vi "Project.vi"() -> ()   [LabVIEW 2023]
uses:
  System.Windows.Forms
  <vilib>/Utility/file.llb/Read Delimited Spreadsheet (string).vi
  <instrlib>/Agilent N934X Series/Public/Configure/Measurement/Configure Measurement (Reflection Measurement).vi
  <instrlib>/Agilent N934X Series/Public/Configure/Measurement/Configure Measurement (Reflection Measurement - DTF).vi
  <instrlib>/Agilent N934X Series/Public/Configure/Configure Frequency (Reflection Measurement - Start Stop).vi
  <vilib>/Utility/file.llb/Write Delimited Spreadsheet (string).vi
  <instrlib>/Agilent N934X Series/Agilent N934X Series.lvlib
panel:
  in  "VISA resource name":refnum<visa-resource-name>
  out "loop#":i32
  in  "jkjk":bool
  out "jkjk":string
  out "jkjk":string
  out "jkjk":string
  in  "jkjk":bool
  in  "Tab Control":T1(tab)
  in  "?":bool
  out "?":string
  out "Step:":i32
  in  "Length of Cable (ft)":dbl=5.0
  in  "?":refnum<k24>(container)
  out "Section:":string
  # "VSWR and Distance to Fault Test"
  # "For a single carrier"
  # "(LBand TX)  +  LBand RX = 2475 MHz"
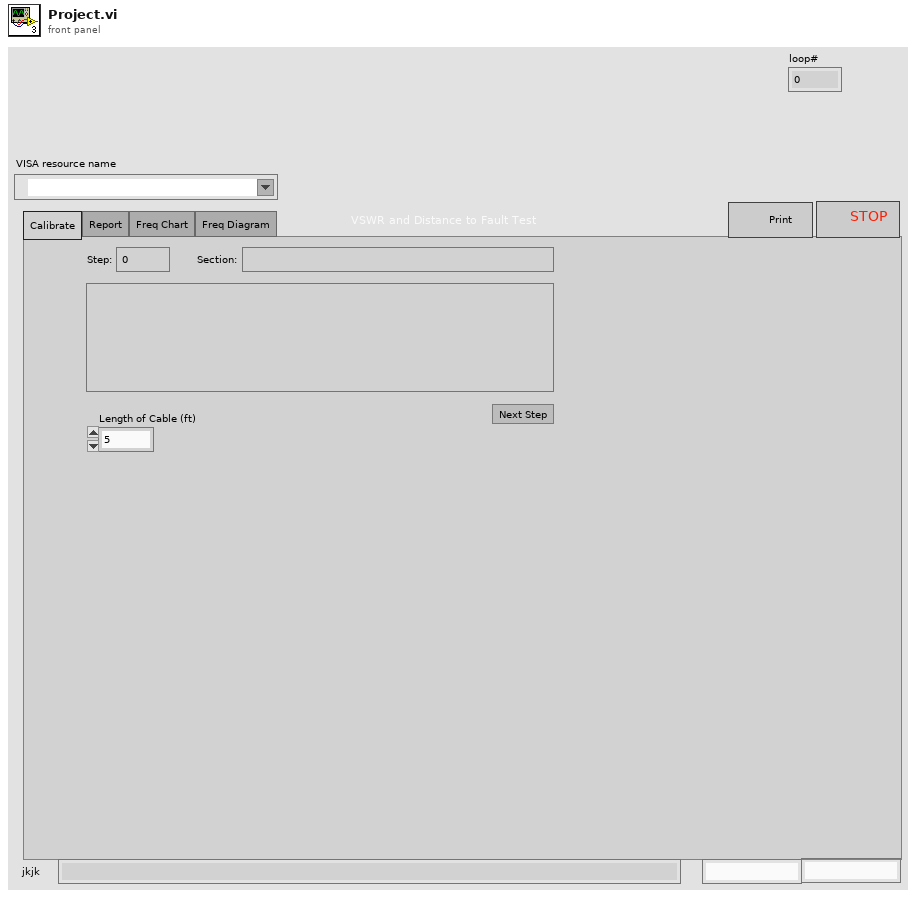
[diagram p1: front panel]
types:
  T1 = enum32{"Calibrate", "Report", "Freq Chart", "Freq Diagram"}
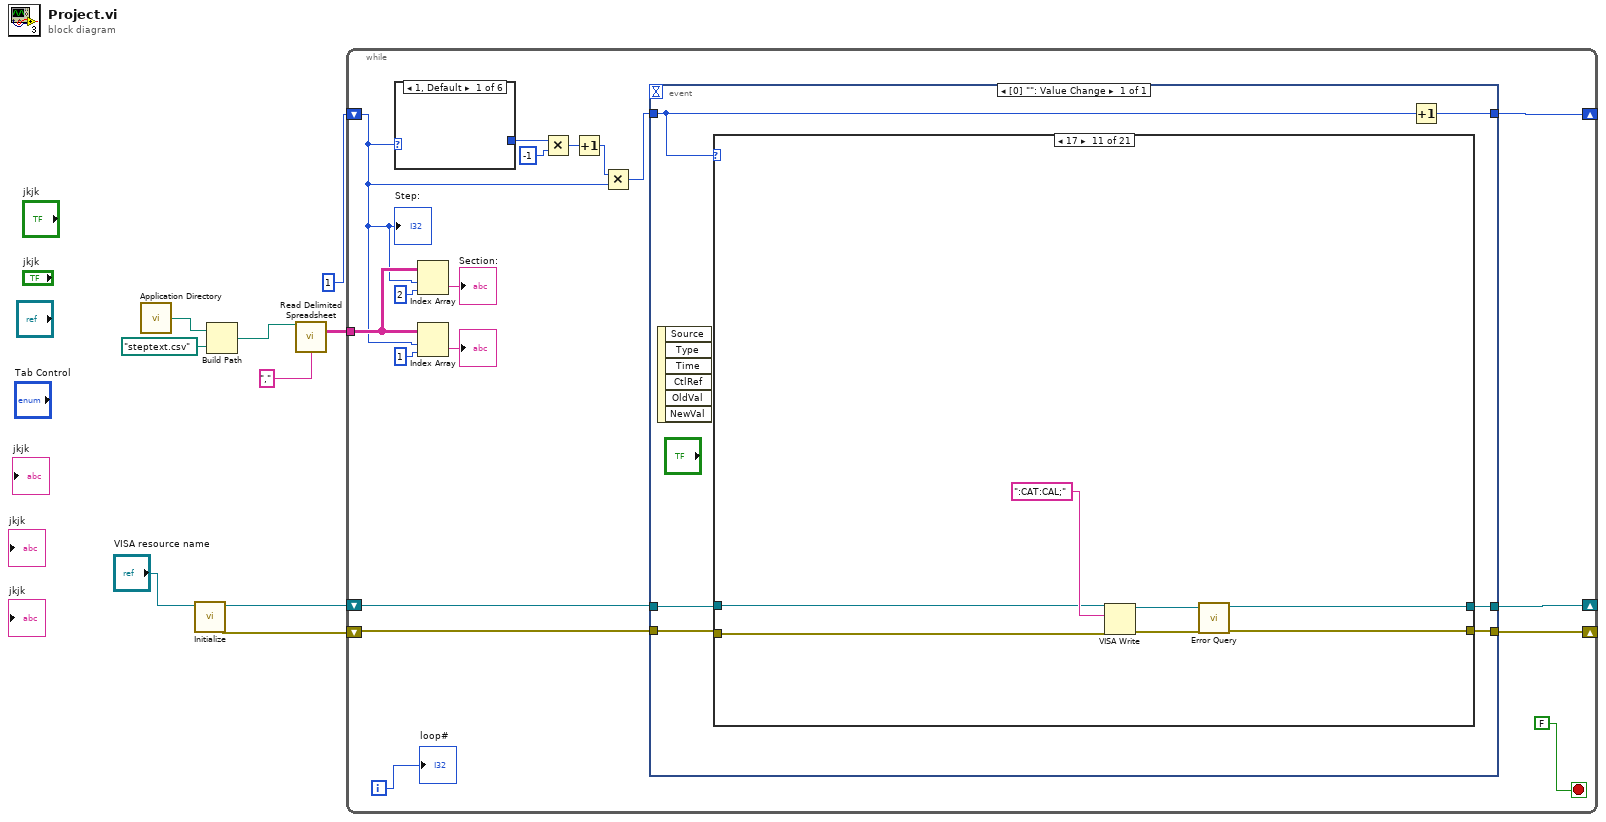
[diagram p0: block diagram]
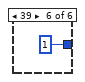
[diagram p6: hidden frame]
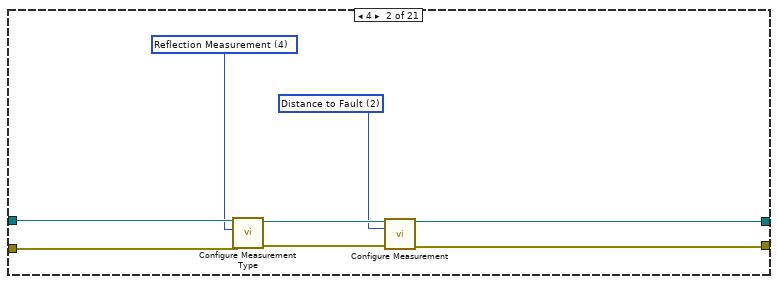
[diagram p8: hidden frame]
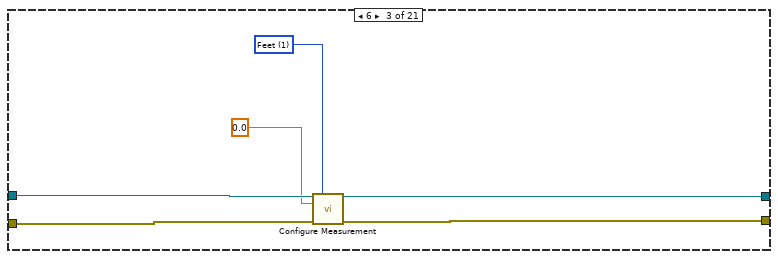
[diagram p9: hidden frame]
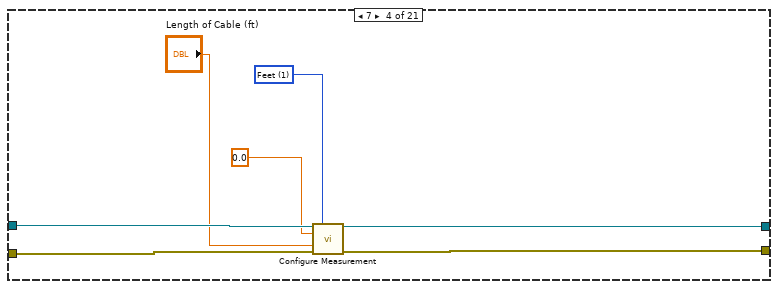
[diagram p10: hidden frame]
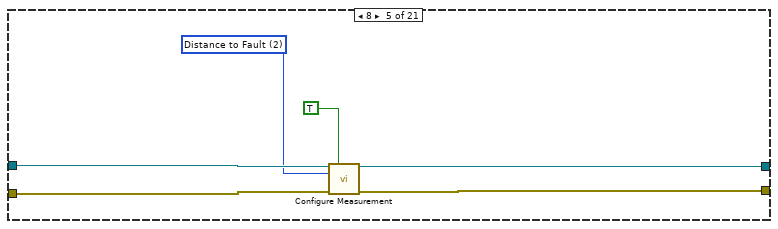
[diagram p11: hidden frame]
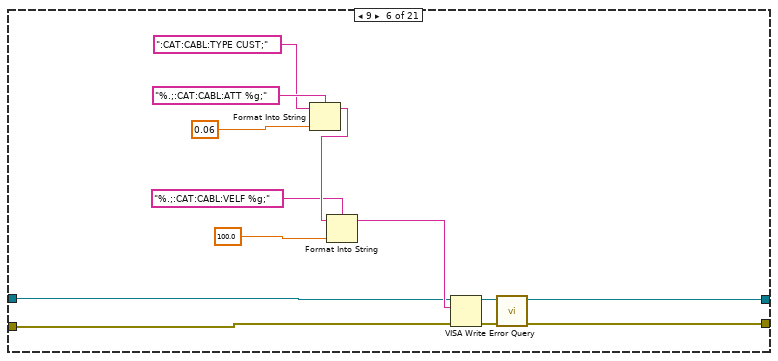
[diagram p12: hidden frame]
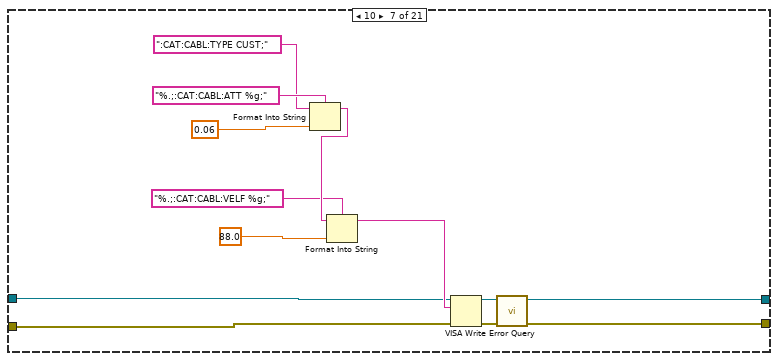
[diagram p13: hidden frame]
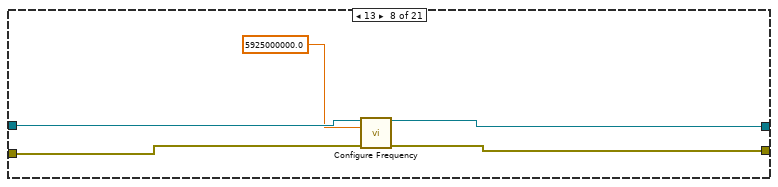
[diagram p14: hidden frame]
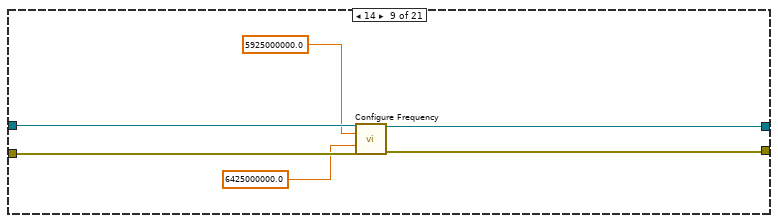
[diagram p15: hidden frame]
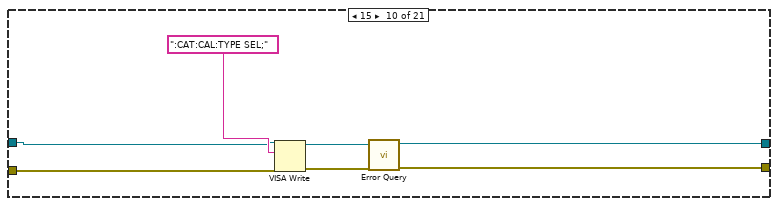
[diagram p16: hidden frame]
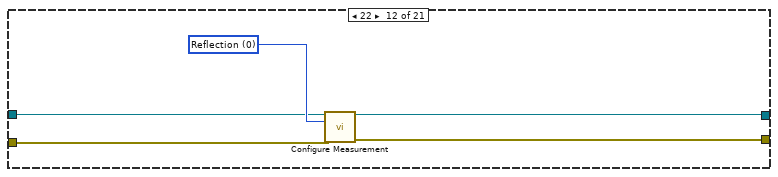
[diagram p17: hidden frame]
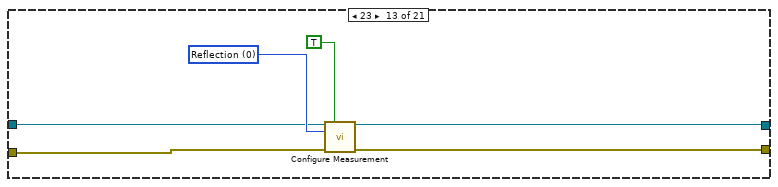
[diagram p18: hidden frame]
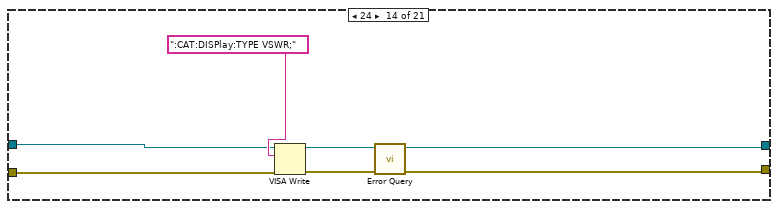
[diagram p19: hidden frame]
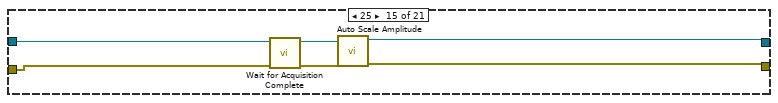
[diagram p20: hidden frame]
diagram:
  n1 = call <vilib>:"Application Directory.vi"() -> ("Application Directory"=w6:path)
  n2 = call <instrlib>:"Initialize.vi"("VISA resource name"="VISA resource name") -> ("error out"=w1:errorcluster, "VISA resource name out"=w2:refnum<visa-resource-name>)  [unwired: 9 in]
  n3 = Build Path(base path=w6, name or relative path=path "steptext.csv") -> (appended path=w4:path)
  n4 = call-poly <vilib>:"Read Delimited Spreadsheet.vi"("file path (dialog if empty)"=w4, "delimiter (\\t)"="," ("delimiter (\\t)")) -> ("all rows"=w7:string[][])  [unwired: 8 in, 5 out]
  n5 = while {
    shift-right: [w25] -> _
    shift-left: 1 -> [w15]
    tunnel: w7 -> [w17]
    shift-right: [w13] -> _
    shift-left: w2 -> [w11]
    shift-right: [w12] -> _
    shift-left: w1 -> [w10]
    i -> [w14]
    stop <- FALSE stop-if-true
    n6 = case shown="1, Default" w15 {
      tunnel: [_ _ _ _ _ 1] -> w24
      frame 1, Default {
      }
      frame 2 {
      }
      frame 3 {
      }
      frame 4 {
      }
      frame 5 {
      }
      frame 39 {
      }
    }
    n7 = Index Array(array=w17, index (row)=w15, index (col)=2) -> (element=→"Section:":string)
    n8 = Index Array(array=w17, index (row)=w15, index (col)=1) -> (element=→"?":string)
    n9 = Multiply(x=w24, y=-1) -> (x*y=w22:i32)
    n10 = Increment(x=w22) -> (x+1=w21:i32)
    n11 = Multiply(x=w21, y=w15) -> (x*y=w26:i32)
    n12 = event shown="[0] \"\": Value Change" {
      selector: _ -> [_]
      dyn-events: _ -> [_]
      timeout: _ -> [_]
      tunnel: w26 -> [w29]
      tunnel: [w34] -> w25
      tunnel: w11 -> [w33]
      tunnel: w10 -> [w31]
      tunnel: [w32] -> w13
      tunnel: [w30] -> w12
      event Value Change {
        n13 = event-data() -> ()  [unwired: 1 in, 6 out]
        n14 = case shown="17" w29 {
          tunnel: w33 -> [w36 w44 w50 w57 w63 w69 w82 w94 w100 w104 w111 w118 w124 w129 w134 w155 w193 w200 w206 w211 w220]
          tunnel: [w36 w38 w47 w54 w60 w66 w79 w91 w97 w101 w109 w116 w122 w127 w137 w141 w195 w198 w204 w215 w218] -> w32
          tunnel: w31 -> [w35 w43 w49 w56 w62 w68 w81 w93 w99 w103 w110 w117 w123 w128 w133 w154 w192 w199 w205 w210 w219]
          tunnel: [w35 w39 w48 w55 w61 w67 w80 w92 w98 w102 w108 w115 w121 w126 w138 w142 w194 w197 w203 w214 w217] -> w30
          frame Default {
          }
          frame 4 {
            w37 = 2 items=["Reflection", "One Port Insertion Loss", "Distance to Fault"] ("Measurement Type (0: Reflection)")
            w42 = 4 items=["Spectrum Analyzer", "Tracking Generator", "Power Meter", "Modulation Analyzer", "Reflection Measurement"] ("Measurement Type (0: Spectrum Analyzer)")
            n15 = call <instrlib>:"Configure Measurement Type.vi"("error in (no error)"=w43, "Measurement Type (0: Spectrum Analyzer)"=w42, "VISA resource name"=w44) -> ("error out"=w40:errorcluster, "VISA resource name out"=w41:refnum<visa-resource-name>)  [unwired: 7 in]
            n16 = call-poly <instrlib>:"Configure Measurement.vi"("VISA resource name"=w41, "Measurement Type (0: Reflection)"=w37, "error in (no error)"=w40) -> ("VISA resource name out"=w38:refnum<visa-resource-name>, "error out"=w39:errorcluster)  [unwired: 11 in]
          }
          frame 6 {
            w46 = 1 items=["Meter", "Feet"] ("Distance Unit (0: Meter)")
            n17 = call-poly <instrlib>:"Configure Measurement.vi"("VISA resource name"=w50, "Distance Unit (0: Meter)"=w46, "Distance Start (0.12 meters)"=0.0, "error in (no error)"=w49) -> ("VISA resource name out"=w47:refnum<visa-resource-name>, "error out"=w48:errorcluster)  [unwired: 10 in]
          }
          frame 7 {
            w53 = 1 items=["Meter", "Feet"] ("Distance Unit (0: Meter)")
            n18 = call-poly <instrlib>:"Configure Measurement.vi"("VISA resource name"=w57, "Distance Unit (0: Meter)"=w53, "Distance Start (0.12 meters)"=0.0, "Distance Stop (0.15 meter)"="Length of Cable (ft)", "error in (no error)"=w56) -> ("VISA resource name out"=w54:refnum<visa-resource-name>, "error out"=w55:errorcluster)  [unwired: 9 in]
          }
          frame 8 {
            w58 = 2 items=["Reflection", "One Port Insertion Loss", "Distance to Fault"] ("Measurement Type (0: Reflection)")
            n19 = call-poly <instrlib>:"Configure Measurement.vi"("VISA resource name"=w63, "Enable IIM (F: Disable)"=TRUE, "Measurement Type (0: Reflection)"=w58, "error in (no error)"=w62) -> ("VISA resource name out"=w60:refnum<visa-resource-name>, "error out"=w61:errorcluster)  [unwired: 10 in]
          }
          frame 9 {
            n20 = Format Into String(format string="%.;:CAT:CABL:ATT %g;", initial string=":CAT:CABL:TYPE CUST;" ("output string"), 0.06 ("input 1")) -> (resulting string=w75:string)  [unwired: 1 in, 1 out]
            n21 = Format Into String(format string="%.;:CAT:CABL:VELF %g;", initial string=w75, 100.0 ("input 1")) -> (resulting string=w76:string)  [unwired: 1 in, 1 out]
            n22 = VISA Write(VISA resource name=w69, write buffer=w76, error in (no error)=w68) -> (VISA resource name out=w73:refnum<visa-resource-name>, error out=w74:errorcluster)  [unwired: 1 out]
            n23 = call <instrlib>:"Error Query.vi"("error in (no error)"=w74, "VISA resource name"=w73) -> ("error out"=w67:errorcluster, "VISA resource name out"=w66:refnum<visa-resource-name>)  [unwired: 6 in, 2 out]
          }
          frame 10 {
            n24 = Format Into String(format string="%.;:CAT:CABL:ATT %g;", initial string=":CAT:CABL:TYPE CUST;" ("output string"), 0.06 ("input 1")) -> (resulting string=w88:string)  [unwired: 1 in, 1 out]
            n25 = Format Into String(format string="%.;:CAT:CABL:VELF %g;", initial string=w88, 88.0 ("input 1")) -> (resulting string=w89:string)  [unwired: 1 in, 1 out]
            n26 = VISA Write(VISA resource name=w82, write buffer=w89, error in (no error)=w81) -> (VISA resource name out=w86:refnum<visa-resource-name>, error out=w87:errorcluster)  [unwired: 1 out]
            n27 = call <instrlib>:"Error Query.vi"("error in (no error)"=w87, "VISA resource name"=w86) -> ("error out"=w80:errorcluster, "VISA resource name out"=w79:refnum<visa-resource-name>)  [unwired: 6 in, 2 out]
          }
          frame 13 {
            n28 = call-poly <instrlib>:"Configure Frequency.vi"("VISA resource name"=w94, "Start Frequency (5E+6 Hz)"=5925000000.0, "error in (no error)"=w93) -> ("VISA resource name out"=w91:refnum<visa-resource-name>, "error out"=w92:errorcluster)  [unwired: 11 in]
          }
          frame 14 {
            n29 = call-poly <instrlib>:"Configure Frequency.vi"("VISA resource name"=w100, "Start Frequency (5E+6 Hz)"=5925000000.0, "Stop Frequency (5E+8 Hz)"=6425000000.0, "error in (no error)"=w99) -> ("VISA resource name out"=w97:refnum<visa-resource-name>, "error out"=w98:errorcluster)  [unwired: 10 in]
          }
          frame 15 {
            n30 = VISA Write(VISA resource name=w104, write buffer=":CAT:CAL:TYPE SEL;", error in (no error)=w103) -> (VISA resource name out=w107:refnum<visa-resource-name>, error out=w106:errorcluster)  [unwired: 1 out]
            n31 = call <instrlib>:"Error Query.vi"("error in (no error)"=w106, "VISA resource name"=w107) -> ("error out"=w102:errorcluster, "VISA resource name out"=w101:refnum<visa-resource-name>)  [unwired: 6 in, 2 out]
          }
          frame 17 {
            n32 = VISA Write(VISA resource name=w111, write buffer=":CAT:CAL;", error in (no error)=w110) -> (VISA resource name out=w114:refnum<visa-resource-name>, error out=w113:errorcluster)  [unwired: 1 out]
            n33 = call <instrlib>:"Error Query.vi"("error in (no error)"=w113, "VISA resource name"=w114) -> ("error out"=w108:errorcluster, "VISA resource name out"=w109:refnum<visa-resource-name>)  [unwired: 6 in, 2 out]
          }
          frame 22 {
            w119 = 0 items=["Reflection", "One Port Insertion Loss", "Distance to Fault"] ("Measurement Type (0: Reflection)")
            n34 = call-poly <instrlib>:"Configure Measurement.vi"("VISA resource name"=w118, "Measurement Type (0: Reflection)"=w119, "error in (no error)"=w117) -> ("VISA resource name out"=w116:refnum<visa-resource-name>, "error out"=w115:errorcluster)  [unwired: 11 in]
          }
          frame 23 {
            w125 = 0 items=["Reflection", "One Port Insertion Loss", "Distance to Fault"] ("Measurement Type (0: Reflection)")
            n35 = call-poly <instrlib>:"Configure Measurement.vi"("VISA resource name"=w124, "Enable IIM (F: Disable)"=TRUE, "Measurement Type (0: Reflection)"=w125, "error in (no error)"=w123) -> ("VISA resource name out"=w122:refnum<visa-resource-name>, "error out"=w121:errorcluster)  [unwired: 10 in]
          }
          frame 24 {
            n36 = VISA Write(VISA resource name=w129, write buffer=":CAT:DISPlay:TYPE VSWR;", error in (no error)=w128) -> (VISA resource name out=w131:refnum<visa-resource-name>, error out=w132:errorcluster)  [unwired: 1 out]
            n37 = call <instrlib>:"Error Query.vi"("error in (no error)"=w132, "VISA resource name"=w131) -> ("error out"=w126:errorcluster, "VISA resource name out"=w127:refnum<visa-resource-name>)  [unwired: 6 in, 2 out]
          }
          frame 25 {
            n38 = call <instrlib>:"Wait for Acquisition Complete.vi"("error in (no error)"=w133, "VISA resource name"=w134) -> ("error out"=w135:errorcluster, "VISA resource name out"=w136:refnum<visa-resource-name>)  [unwired: 8 in]
            n39 = call <instrlib>:"Auto Scale Amplitude.vi"("error in (no error)"=w135, "VISA resource name"=w136) -> ("error out"=w138:errorcluster, "VISA resource name out"=w137:refnum<visa-resource-name>)  [unwired: 8 in]
          }
          frame 26 {
            # "init file, if doesn't exist"
            # "bruh"
            n40 = VISA Write(VISA resource name=w155, write buffer=":CALC:MARK:AOFF", error in (no error)=w154) -> (VISA resource name out=w168:refnum<visa-resource-name>, error out=w169:errorcluster)  [unwired: 1 out]
            n41 = call <vilib>:"Application Directory.vi"() -> ("Application Directory"=w164:path)
            n42 = call <instrlib>:"Configure Marker Reflection Measurement.vi"("Enable Continuous Peak (F: Disable)"=TRUE, "error in (no error)"=w169, "VISA resource name"=w168) -> ("error out"=w177:errorcluster, "VISA resource name out"=w179:refnum<visa-resource-name>)  [unwired: 7 in]
            n43 = Build Path(base path=w164, name or relative path=path "history_vswr.csv") -> (appended path=w152:path)
            n44 = Format Into String(format string=":CALC:MARK%d:X?;", 1 ("input 1")) -> (resulting string=w171:string)  [unwired: 2 in, 1 out]
            n45 = call <vilib>:"Check if File or Folder Exists.vi"("path"=w152) -> ("file or folder exists?"=w149:bool, "dup path"=w151:path)  [unwired: 8 in, 1 out]
            n46 = VISA Write(VISA resource name=w179, write buffer=w171, error in (no error)=w177) -> (VISA resource name out=w172:refnum<visa-resource-name>, error out=w173:errorcluster)  [unwired: 1 out]
            n47 = VISA Read(VISA resource name=w172, byte count=u32 1000, error in (no error)=w173) -> (VISA resource name out=w174:refnum<visa-resource-name>, read buffer=w176:string, error out=w175:errorcluster)  [unwired: 1 out]
            n48 = case shown="False" w149 {
              tunnel: w151 -> [w184 w191]
              tunnel: [w183 w191] -> w150
              frame False {
                n49 = Build Array("date" ("element"), "time" ("element"), "freq (mhz)" ("element"), "peak vswr" ("element"), "trace" ("element")) -> (w190:string[])
                n50 = call-poly <vilib>:"Write Delimited Spreadsheet.vi"("file path (dialog if empty)"=w184, "1D data"=w190, "delimiter (\\t)"="," ("delimiter (\\t)")) -> ("new file path (Not A Path if cancelled)"=w183:path)  [unwired: 11 in, 1 out]
              }
              frame True {
              }
            }
            n51 = Scan From String(format string="%.;%g", input string=w176) -> (output 1=w146:dbl)  [unwired: 3 in, 3 out]
            n52 = call <instrlib>:"Error Query.vi"("error in (no error)"=w175, "VISA resource name"=w174) -> ("error out"=w178:errorcluster, "VISA resource name out"=w180:refnum<visa-resource-name>)  [unwired: 6 in, 2 out]
            n53 = call <instrlib>:"Query Marker.vi"("error in (no error)"=w178, "VISA resource name"=w180) -> ("error out"=w143:errorcluster, "Y Value"=w170:dbl, "VISA resource name out"=w144:refnum<visa-resource-name>)  [unwired: 7 in]
            n54 = Divide(x=w146, y=1000000.0) -> (x/y=w145:dbl)
            n55 = call <instrlib>:"Read Trace (Reflection Measurement).vi"("error in (no error)"=w143, "VISA resource name"=w144) -> ("error out"=w142:errorcluster, "Trace Data"=w139:dbl[], "VISA resource name out"=w141:refnum<visa-resource-name>)  [unwired: 7 in]
            n56 = Get Date/Time String() -> (date string=w166:string, time string=w167:string)  [unwired: 3 in]
            n57 = Number To Fractional String(number=w145) -> (F-format string=w148:string)  [unwired: 3 in]
            n58 = Number To Fractional String(number=w170) -> (F-format string=w181:string)  [unwired: 3 in]
            n59 = Number To Fractional String(number=w139) -> (F-format string=w140:string[])  [unwired: 3 in]
            n60 = Build Array (concatenate)(w166, w167, w148, w181, w140) -> (w165:string[])
            n61 = call-poly <vilib>:"Write Delimited Spreadsheet.vi"("file path (dialog if empty)"=w150, "1D data"=w165, "append to file? (new file:F)"=TRUE, "delimiter (\\t)"="," ("delimiter (\\t)")) -> ()  [unwired: 10 in, 2 out]
          }
          frame 31 {
            w196 = 2 items=["Reflection", "One Port Insertion Loss", "Distance to Fault"] ("Measurement Type (0: Reflection)")
            n62 = call-poly <instrlib>:"Configure Measurement.vi"("VISA resource name"=w193, "Measurement Type (0: Reflection)"=w196, "error in (no error)"=w192) -> ("VISA resource name out"=w195:refnum<visa-resource-name>, "error out"=w194:errorcluster)  [unwired: 11 in]
          }
          frame 32 {
            w202 = 2 items=["Reflection", "One Port Insertion Loss", "Distance to Fault"] ("Measurement Type (0: Reflection)")
            n63 = call-poly <instrlib>:"Configure Measurement.vi"("VISA resource name"=w200, "Enable IIM (F: Disable)"=FALSE, "Measurement Type (0: Reflection)"=w202, "error in (no error)"=w199) -> ("VISA resource name out"=w198:refnum<visa-resource-name>, "error out"=w197:errorcluster)  [unwired: 10 in]
          }
          frame 33 {
            n64 = VISA Write(VISA resource name=w206, write buffer=":CAT:DISPlay:TYPE VSWR;", error in (no error)=w205) -> (VISA resource name out=w208:refnum<visa-resource-name>, error out=w209:errorcluster)  [unwired: 1 out]
            n65 = call <instrlib>:"Error Query.vi"("error in (no error)"=w209, "VISA resource name"=w208) -> ("error out"=w203:errorcluster, "VISA resource name out"=w204:refnum<visa-resource-name>)  [unwired: 6 in, 2 out]
          }
          frame 34 {
            n66 = call <instrlib>:"Wait for Acquisition Complete.vi"("error in (no error)"=w210, "VISA resource name"=w211) -> ("error out"=w212:errorcluster, "VISA resource name out"=w213:refnum<visa-resource-name>)  [unwired: 8 in]
            n67 = call <instrlib>:"Auto Scale Amplitude.vi"("error in (no error)"=w212, "VISA resource name"=w213) -> ("error out"=w214:errorcluster, "VISA resource name out"=w215:refnum<visa-resource-name>)  [unwired: 8 in]
          }
          frame 37 {
            # "init file, if doesn't exist"
            # "bruh"
            n68 = VISA Write(VISA resource name=w220, write buffer=":CALC:MARK:AOFF", error in (no error)=w219) -> (VISA resource name out=w243:refnum<visa-resource-name>, error out=w244:errorcluster)  [unwired: 1 out]
            n69 = call <vilib>:"Application Directory.vi"() -> ("Application Directory"=w239:path)
            n70 = call <instrlib>:"Configure Marker Reflection Measurement.vi"("Enable Continuous Peak (F: Disable)"=TRUE, "error in (no error)"=w244, "VISA resource name"=w243) -> ("error out"=w252:errorcluster, "VISA resource name out"=w254:refnum<visa-resource-name>)  [unwired: 7 in]
            n71 = Build Path(base path=w239, name or relative path=path "history_dtf.csv") -> (appended path=w229:path)
            n72 = Format Into String(format string=":CALC:MARK%d:X?;", 1 ("input 1")) -> (resulting string=w246:string)  [unwired: 2 in, 1 out]
            n73 = call <vilib>:"Check if File or Folder Exists.vi"("path"=w229) -> ("file or folder exists?"=w226:bool, "dup path"=w228:path)  [unwired: 8 in, 1 out]
            n74 = VISA Write(VISA resource name=w254, write buffer=w246, error in (no error)=w252) -> (VISA resource name out=w247:refnum<visa-resource-name>, error out=w248:errorcluster)  [unwired: 1 out]
            n75 = VISA Read(VISA resource name=w247, byte count=u32 1000, error in (no error)=w248) -> (VISA resource name out=w249:refnum<visa-resource-name>, read buffer=w251:string, error out=w250:errorcluster)  [unwired: 1 out]
            n76 = case shown="False" w226 {
              tunnel: w228 -> [w259 w266]
              tunnel: [w258 w266] -> w227
              frame False {
                n77 = Build Array("date" ("element"), "time" ("element"), "dist (ft)" ("element"), "peak vswr" ("element"), "trace" ("element")) -> (w265:string[])
                n78 = call-poly <vilib>:"Write Delimited Spreadsheet.vi"("file path (dialog if empty)"=w259, "1D data"=w265, "delimiter (\\t)"="," ("delimiter (\\t)")) -> ("new file path (Not A Path if cancelled)"=w258:path)  [unwired: 11 in, 1 out]
              }
              frame True {
              }
            }
            n79 = Scan From String(format string="%.;%g", input string=w251) -> (output 1=w216:dbl)  [unwired: 3 in, 3 out]
            n80 = call <instrlib>:"Error Query.vi"("error in (no error)"=w250, "VISA resource name"=w249) -> ("error out"=w253:errorcluster, "VISA resource name out"=w255:refnum<visa-resource-name>)  [unwired: 6 in, 2 out]
            n81 = call <instrlib>:"Query Marker.vi"("error in (no error)"=w253, "VISA resource name"=w255) -> ("error out"=w223:errorcluster, "Y Value"=w245:dbl, "VISA resource name out"=w224:refnum<visa-resource-name>)  [unwired: 7 in]
            n82 = call <instrlib>:"Read Trace (Reflection Measurement).vi"("error in (no error)"=w223, "VISA resource name"=w224) -> ("error out"=w217:errorcluster, "Trace Data"=w221:dbl[], "VISA resource name out"=w218:refnum<visa-resource-name>)  [unwired: 7 in]
            n83 = Get Date/Time String() -> (date string=w241:string, time string=w242:string)  [unwired: 3 in]
            n84 = Number To Fractional String(number=w216) -> (F-format string=w225:string)  [unwired: 3 in]
            n85 = Number To Fractional String(number=w245) -> (F-format string=w256:string)  [unwired: 3 in]
            n86 = Number To Fractional String(number=w221) -> (F-format string=w222:string[])  [unwired: 3 in]
            n87 = Build Array (concatenate)(w241, w242, w225, w256, w222) -> (w240:string[])
            n88 = call-poly <vilib>:"Write Delimited Spreadsheet.vi"("file path (dialog if empty)"=w227, "1D data"=w240, "append to file? (new file:F)"=TRUE, "delimiter (\\t)"="," ("delimiter (\\t)")) -> ()  [unwired: 10 in, 2 out]
          }
        }
        n89 = Increment(x=w29) -> (x+1=w34:i32)
      }
    }
    "Step:" <- w15
    "loop#" <- w14
  }
